vi "get_wvfm_graph_cursor_psoitions.vi"(7 "Difference Trace":refnum<vi>) -> (4 "X Pos Array":dbl[](array[numeric]), 15 "Y Pos Array":dbl[](array[numeric]))   [LabVIEW 2020]
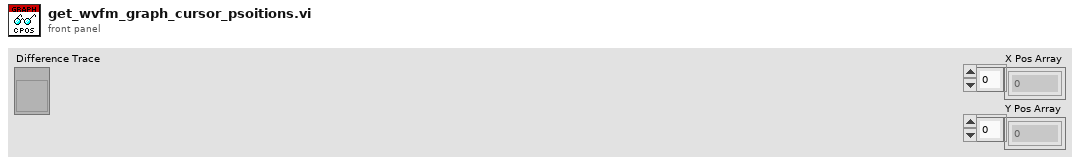
[diagram p1: front panel]
types:
  T1 = typedef "LVCursorListTypeDef.ctl" = cluster{"Name":string, "Color":u32, "Style":u8, "Point Style":u8, "Name Visible":bool, "Allow Drag":bool, "Cursor Mode":u32, "Plot":i32, "Index":i32, "Position":cluster{"X":dbl, "Y":dbl}, "X Scale":u32, "Y Scale":u32, "Watch Plots":i32[], "Watch All Plots":bool, "Plot Area":i32, "Label Offset":cluster{"X":dbl, "Y":dbl}}[]
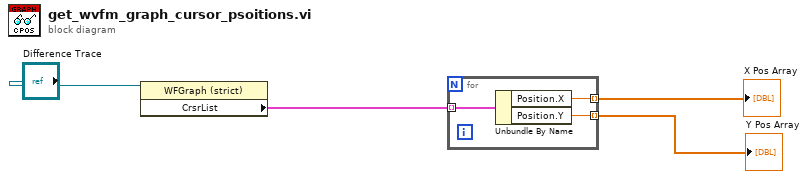
[diagram p0: block diagram]
diagram:
  n1 = property class="WFGraph (strict)"(reference="Difference Trace") -> ("CrsrList"=w4:T1)  [unwired: 1 in, 2 out]
  n2 = for {
    tunnel: w4 -> [w7] mode=indexing
    tunnel: [w6] -> w3 mode=indexing
    tunnel: [w5] -> w2 mode=indexing
    n3 = Unbundle By Name(w7) -> ("Position.X"=w6:dbl, "Position.Y"=w5:dbl)
  }
  "X Pos Array" <- w3
  "Y Pos Array" <- w2
